vi "serial_cycle_thread.vi"() -> ()   [LabVIEW 2020]
doc: "该模板用于创建生产者／消费者模式的应用程序，以事件驱动的方式，生成队列中的项。如需通过响应事件实现代码的异步执行，同时不影响用户界面的响应速度，可考虑用该模式替代“用户界面事件处理器”模式。"
uses:
  <vilib>/Instr/_visa.llb/VISA Set IO Buffer Mask.ctl
  <vilib>/Instr/_visa.llb/VISA Configure Serial Port (Instr).vi
panel:
  in  "写入缓冲区":string="~\u00010000@SCNTRG1;\u0003"
  out "标准码词":string
  out "数据读取时间2":u32
  out "读取的数据":string
  in  "开等待(ms)2":u32
  in  "VISA资源名称2":refnum<visa-resource-name>
  in  "VISA资源名称 3":refnum<visa-resource-name>
  in  "开等待(ms)3":u32
  out "数据读取时间3":u32
  out "读取的数据3":string
  in  "开等待(ms)1":u32
  out "数据读取时间":u32
  out "读取的数据":string
  in  "VISA资源名称":refnum<visa-resource-name>
  in  "读取标准码词":bool
  in  "压缩机":bool
  in  "臭氧":bool
  in  "开始测试":bool
  in  "风机":bool
  in  "继电器调试":bool
  in  "打开开关":bool
  in  "串口资源":refnum<visa-resource-name>
  in  "stop":bool caption="停止"
  out "错误输出":errorcluster
  out "error out":errorcluster caption="继电器板错误输入输出"
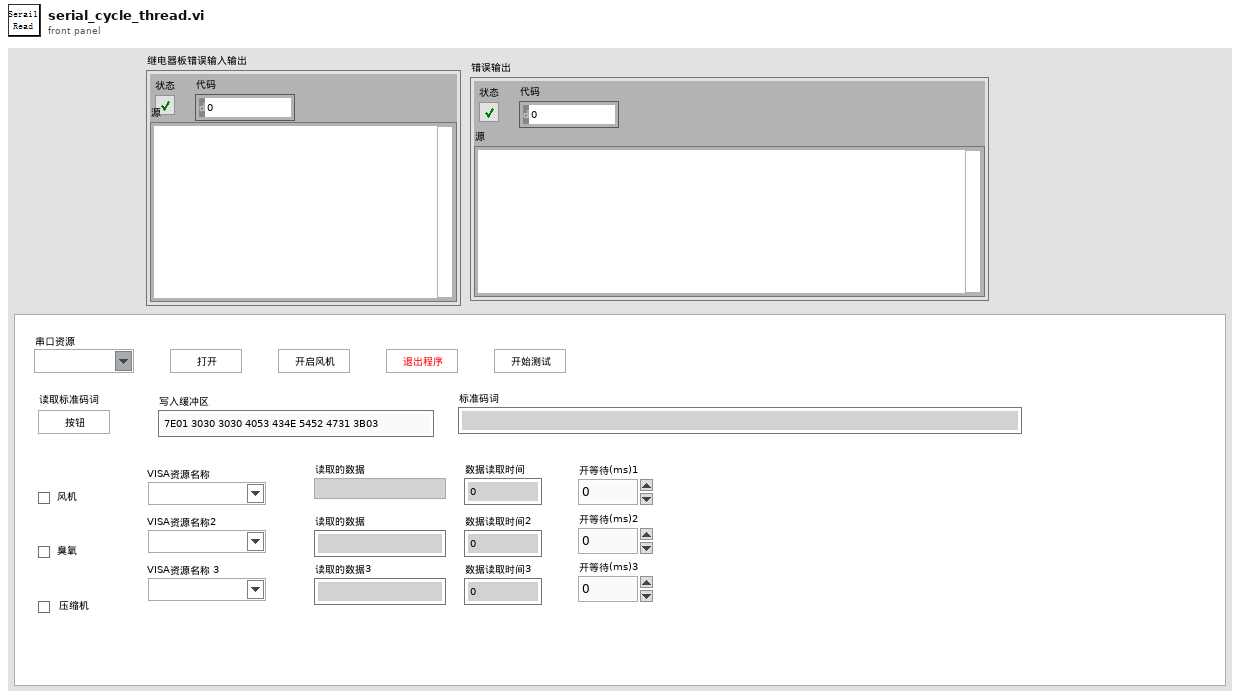
[diagram p1: front panel]
types:
  T1 = typedef "VISA Set IO Buffer Mask.ctl" = u16
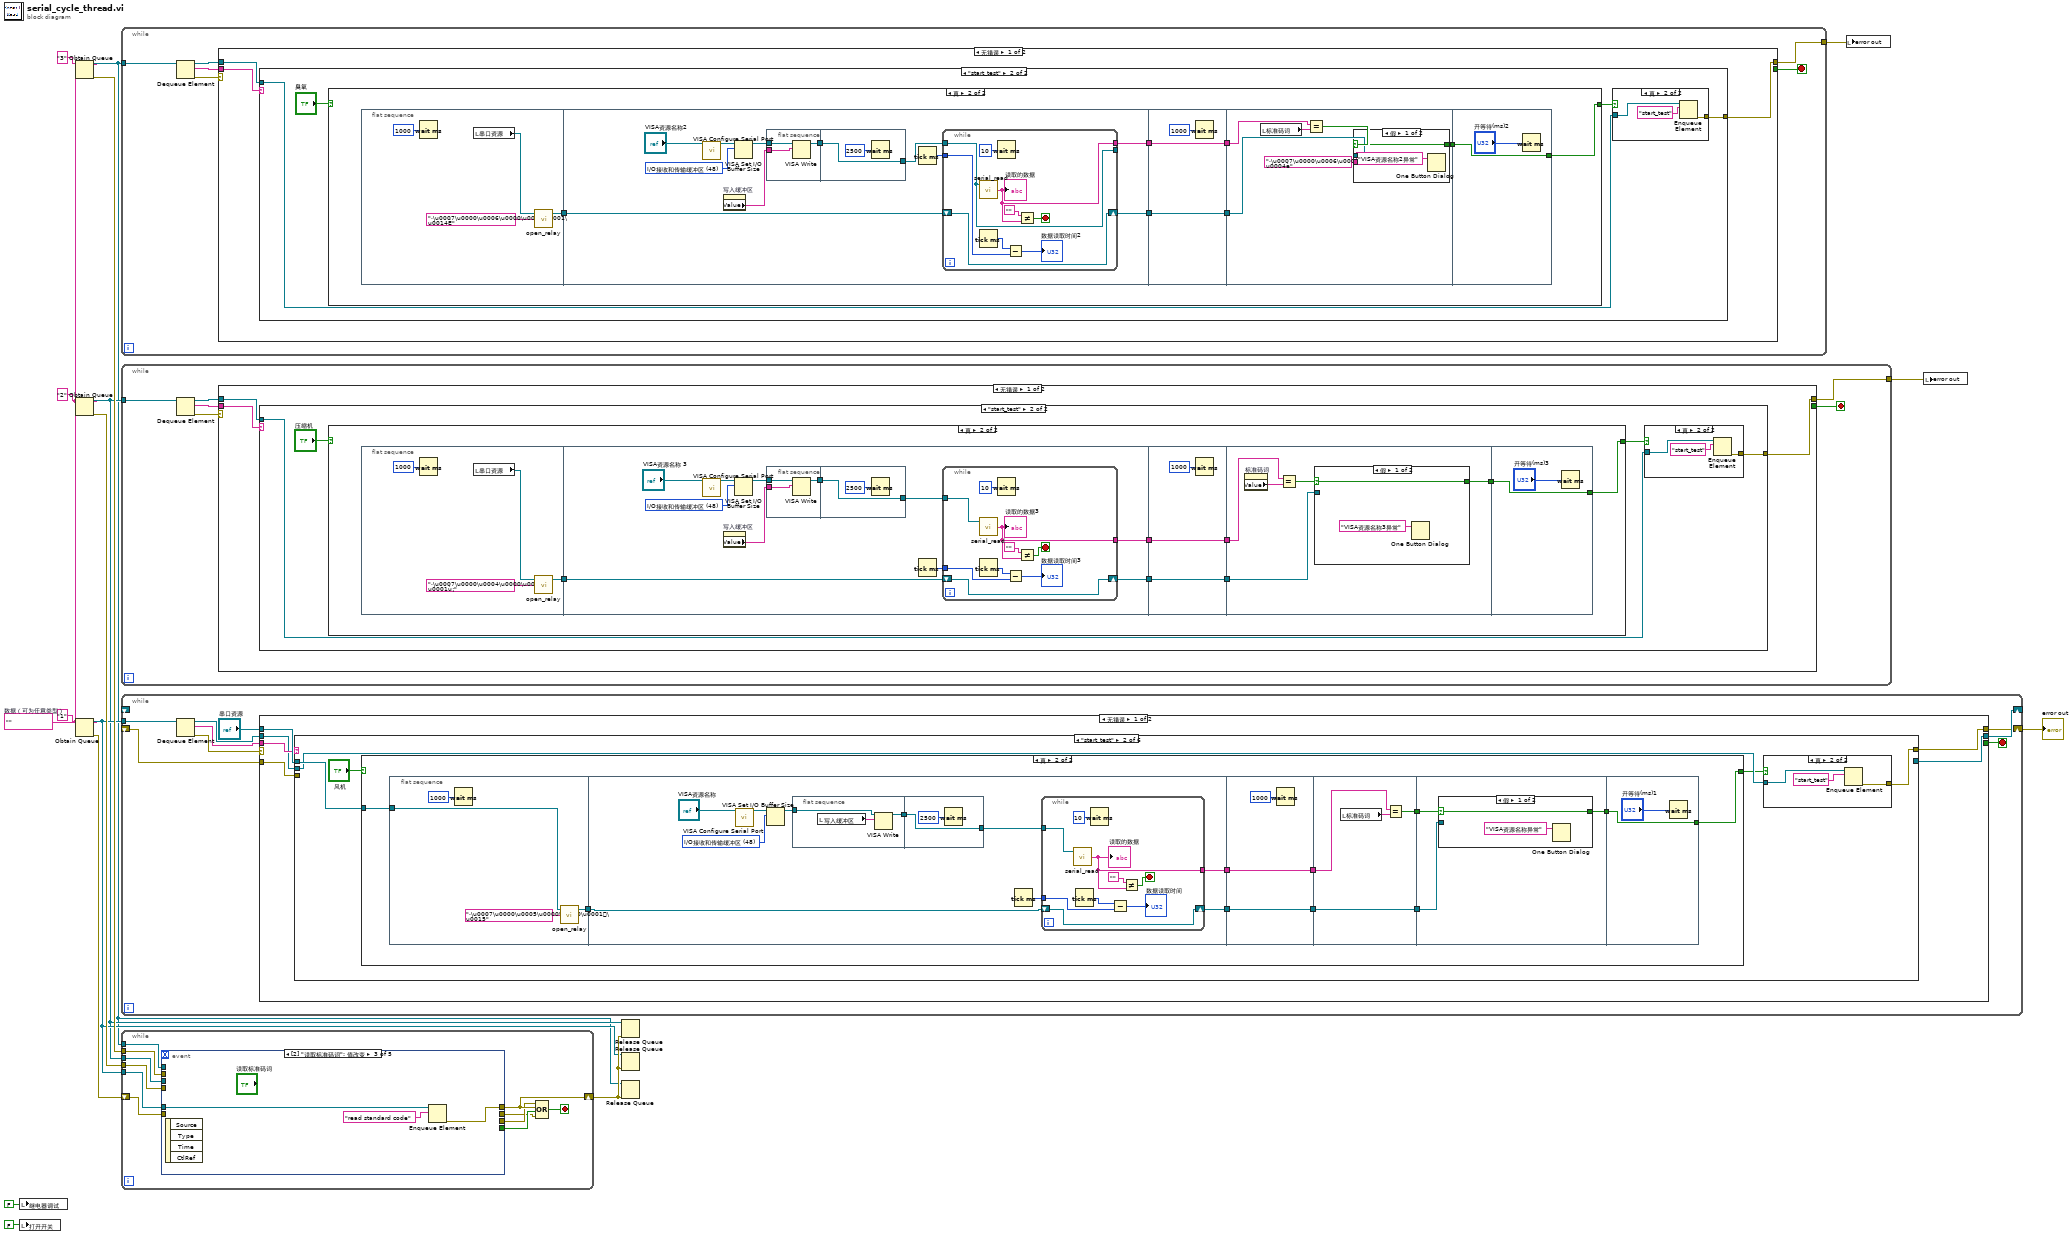
[diagram p0: block diagram]
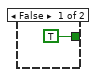
[diagram p4: hidden frame]
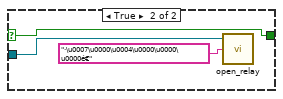
[diagram p5: hidden frame]
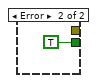
[diagram p6: hidden frame]
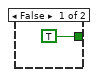
[diagram p9: hidden frame]
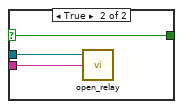
[diagram p10: hidden frame]
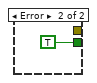
[diagram p11: hidden frame]
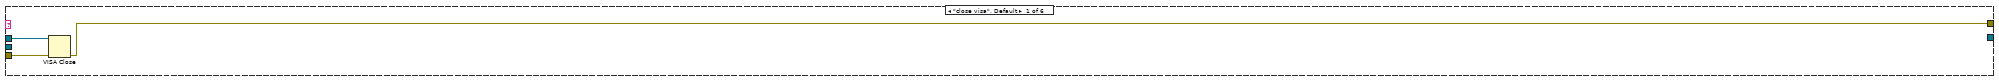
[diagram p12: hidden frame]
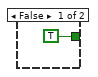
[diagram p14: hidden frame]
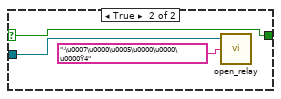
[diagram p15: hidden frame]
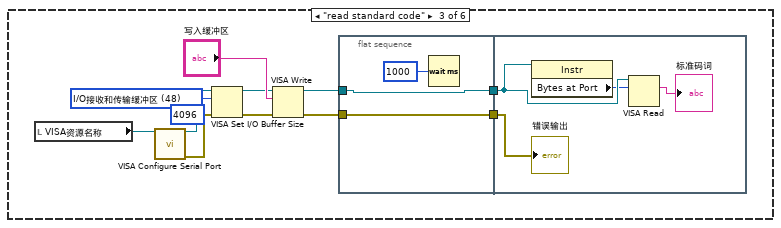
[diagram p16: hidden frame]
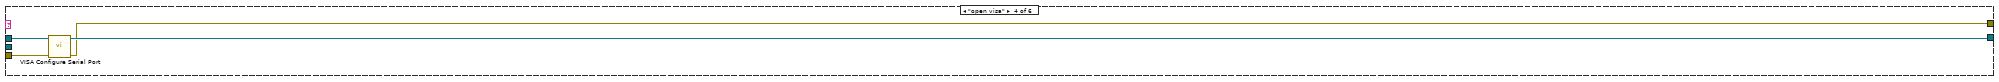
[diagram p17: hidden frame]
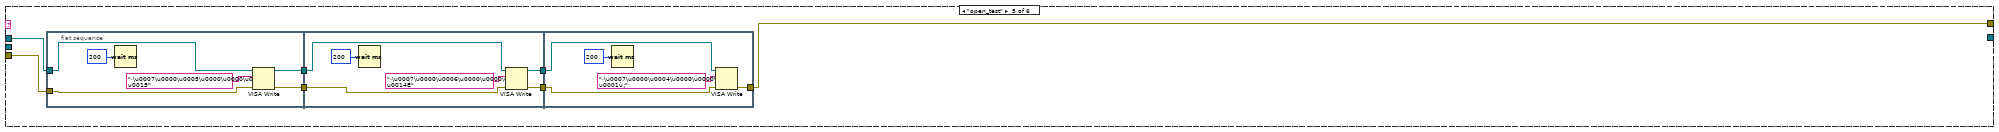
[diagram p18: hidden frame]
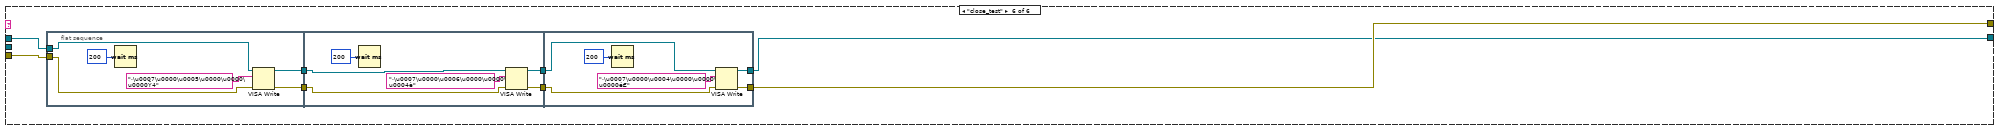
[diagram p19: hidden frame]
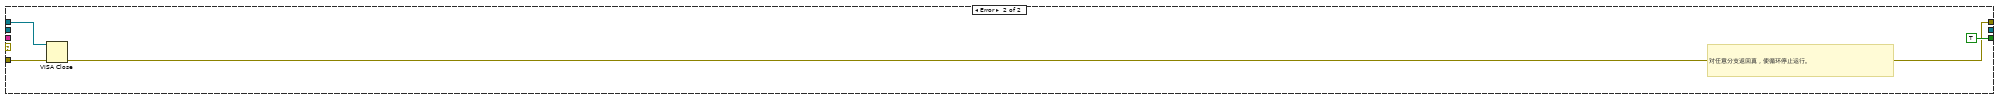
[diagram p20: hidden frame]
diagram:
  w12 = ""  # 数据（可为任意类型）
  n1 = local write "继电器调试"(FALSE ("继电器调试")) -> ()
  n2 = local write "打开开关"(FALSE ("打开开关")) -> ()
  n3 = Obtain Queue(name (unnamed)="3" ("名称（未命名）"), element data type=w12) -> (queue out=w3:refnum<queue>, error out=w11:errorcluster)  [unwired: 3 in, 1 out]
  n4 = Obtain Queue(name (unnamed)="2" ("名称（未命名）"), element data type=w12) -> (queue out=w4:refnum<queue>, error out=w10:errorcluster)  [unwired: 3 in, 1 out]
  n5 = Obtain Queue(name (unnamed)="1" ("名称（未命名）"), element data type=w12) -> (queue out=w8:refnum<queue>, error out=w16:errorcluster)  [unwired: 3 in, 1 out]
  n6 = while {
    tunnel: w3 -> [w19]
    tunnel: [w18] -> w1
    stop <- w20 stop-if-true
    n7 = Dequeue Element(queue=w19) -> (queue out=w17:refnum<queue>, element=w21:string, error out=w22:errorcluster)  [unwired: 2 in, 1 out]
    n8 = case shown="无错误" w22 {
      tunnel: w21 -> [w25 _]
      tunnel: [_ TRUE] -> w20
      tunnel: [w24 _] -> w18
      tunnel: w17 -> [w23 _]
      frame No Error {
        n9 = case shown="\"start_test\"" w25 {
          tunnel: [_ w27] -> w24
          tunnel: w23 -> [_ w26]
          frame "假", Default {
          }
          frame "start_test" {
            n10 = case shown="真" "臭氧" {
              tunnel: [TRUE w37] -> w28
              frame False {
              }
              frame True {
                n11 = flat-sequence {
                  tunnel: [w43] -> w40
                  tunnel: w40 -> [w55]
                  tunnel: [w54] -> w39
                  tunnel: [w45] -> w35
                  tunnel: w39 -> [w72]
                  tunnel: [w72] -> w38
                  tunnel: [w70] -> w36
                  tunnel: w35 -> [w70]
                  tunnel: w38 -> [w74]
                  tunnel: w36 -> [w78]
                  tunnel: [w73] -> w34
                  tunnel: [w84] -> w37
                  tunnel: w34 -> [w84]
                  frame #0 {
                    n12 = Wait (ms)(milliseconds to wait=u32 1000 ("等待时间（毫秒）")) -> ()  [unwired: 1 out]
                    n13 = local read "串口资源"() -> (w41:refnum<visa-resource-name>)
                    n14 = call "open_relay.vi"("写入缓冲区"="·\u0007\u0000\u0006\u0000\u0000\u0001\u0014É", "VISA资源名称"=w41) -> ("VISA资源名称输出"=w43:refnum<visa-resource-name>)  [unwired: 1 in, 2 out]
                  }
                  frame #1 {
                    w50 = T1 48 items=["I/O接收缓冲区"=16, "I/O传输缓冲区"=32, "I/O接收和传输缓冲区"=48] ("Mask")
                    n15 = call-poly "VISA Configure Serial Port"("VISA resource name"="VISA资源名称2") -> ("VISA resource name out"=w51:refnum<visa-resource-name>)  [unwired: 13 in, 1 out]
                    n16 = property on="写入缓冲区" class="Str"() -> ("Value"=w49:string)  [unwired: 2 in, 2 out]
                    n17 = VISA Set I/O Buffer Size(VISA resource name=w51, mask (16)=w50) -> (VISA resource name out=w48:refnum<visa-resource-name>)  [unwired: 2 in, 1 out]
                    n18 = flat-sequence {
                      tunnel: w49 -> [w58]
                      tunnel: w48 -> [w57]
                      tunnel: [w56] -> w46
                      tunnel: [w60] -> w47
                      tunnel: w46 -> [w60]
                      frame #0 {
                        n19 = VISA Write(VISA resource name=w57, write buffer=w58) -> (VISA resource name out=w56:refnum<visa-resource-name>)  [unwired: 1 in, 2 out]
                      }
                      frame #1 {
                        n20 = Wait (ms)(milliseconds to wait=u32 2500 ("等待时间（毫秒）")) -> ()  [unwired: 1 out]
                      }
                    }
                    n21 = Tick Count (ms)() -> (millisecond timer value=w53:u32)
                    n22 = while {
                      shift-right: [w66] -> w54
                      shift-left: w55 -> [w66]
                      tunnel: [w62] -> _
                      tunnel: w53 -> [w64]
                      tunnel: w47 -> [w62]
                      tunnel: [w61] -> w45
                      stop <- w68 stop-if-true
                      n23 = call "serial_read.vi"("VISA资源名称"=w62) -> ("读取缓冲区"=w61:string)  [unwired: 2 in, 2 out]
                      "读取的数据" <- w61
                      n24 = Tick Count (ms)() -> (millisecond timer value=w65:u32)
                      n25 = Wait (ms)(milliseconds to wait=u32 10 ("等待时间（毫秒）")) -> ()  [unwired: 1 out]
                      n26 = Subtract(x=w65, y=w64) -> (x-y=→"数据读取时间2":u32)
                      n27 = Not Equal?(x="", y=w61) -> (x != y?=w68:bool)
                    }
                  }
                  frame #2 {
                    n28 = Wait (ms)(milliseconds to wait=u32 1000 ("等待时间（毫秒）")) -> ()  [unwired: 1 out]
                  }
                  frame #3 {
                    n29 = local read "标准码词"() -> (w77:string)
                    n30 = Equal?(x=w78, y=w77) -> (x = y?=w76:bool)
                    n31 = case shown="假" w76 {
                      selector: w76 -> [w80 w81]
                      tunnel: "·\u0007\u0000\u0006\u0000\u0000\u0000\u0004è" ("写入缓冲区") -> [_ w83]
                      tunnel: w74 -> [_ w82]
                      tunnel: [w80 w81] -> w73
                      frame False {
                        n32 = One Button Dialog(message="VISA资源名称2异常" ("消息")) -> ()  [unwired: 1 in, 1 out]
                      }
                      frame True {
                        n33 = call "open_relay.vi"("写入缓冲区"=w83, "VISA资源名称"=w82) -> ()  [unwired: 1 in, 3 out]
                      }
                    }
                  }
                  frame #4 {
                    n34 = Wait (ms)(milliseconds to wait="开等待(ms)2") -> ()  [unwired: 1 out]
                  }
                }
              }
            }
            n35 = case shown="真" w28 {
              tunnel: [_ w31] -> w27
              tunnel: w26 -> [_ w30]
              frame False {
              }
              frame True {
                n36 = Enqueue Element(queue=w30, element="start_test" ("元素")) -> (error out=w31:errorcluster)  [unwired: 2 in, 2 out]
              }
            }
          }
        }
      }
      frame Error {
      }
    }
  }
  n37 = while {
    tunnel: w4 -> [w89]
    tunnel: [w88] -> w2
    stop <- w90 stop-if-true
    n38 = Dequeue Element(queue=w89) -> (queue out=w87:refnum<queue>, element=w91:string, error out=w92:errorcluster)  [unwired: 2 in, 1 out]
    n39 = case shown="无错误" w92 {
      tunnel: w91 -> [w95 _]
      tunnel: [_ TRUE] -> w90
      tunnel: [w94 _] -> w88
      tunnel: w87 -> [w93 _]
      frame No Error {
        n40 = case shown="\"start_test\"" w95 {
          tunnel: [_ w97] -> w94
          tunnel: w93 -> [_ w96]
          frame "假", Default {
          }
          frame "start_test" {
            n41 = case shown="真" "压缩机" {
              tunnel: [TRUE w107] -> w98
              frame False {
              }
              frame True {
                n42 = flat-sequence {
                  tunnel: [w113] -> w110
                  tunnel: w110 -> [w125]
                  tunnel: [w124] -> w109
                  tunnel: [w115] -> w105
                  tunnel: w109 -> [w142]
                  tunnel: [w142] -> w108
                  tunnel: [w140] -> w106
                  tunnel: w105 -> [w140]
                  tunnel: w108 -> [w144]
                  tunnel: w106 -> [w147]
                  tunnel: [w143] -> w104
                  tunnel: [w153] -> w107
                  tunnel: w104 -> [w153]
                  frame #0 {
                    n43 = Wait (ms)(milliseconds to wait=u32 1000 ("等待时间（毫秒）")) -> ()  [unwired: 1 out]
                    n44 = local read "串口资源"() -> (w111:refnum<visa-resource-name>)
                    n45 = call "open_relay.vi"("写入缓冲区"="·\u0007\u0000\u0004\u0000\u0000\u0001ù¡", "VISA资源名称"=w111) -> ("VISA资源名称输出"=w113:refnum<visa-resource-name>)  [unwired: 1 in, 2 out]
                  }
                  frame #1 {
                    w120 = T1 48 items=["I/O接收缓冲区"=16, "I/O传输缓冲区"=32, "I/O接收和传输缓冲区"=48] ("Mask")
                    n46 = call-poly "VISA Configure Serial Port"("VISA resource name"="VISA资源名称 3") -> ("VISA resource name out"=w121:refnum<visa-resource-name>)  [unwired: 13 in, 1 out]
                    n47 = property on="写入缓冲区" class="Str"() -> ("Value"=w117:string)  [unwired: 2 in, 2 out]
                    n48 = VISA Set I/O Buffer Size(VISA resource name=w121, mask (16)=w120) -> (VISA resource name out=w119:refnum<visa-resource-name>)  [unwired: 2 in, 1 out]
                    n49 = flat-sequence {
                      tunnel: w119 -> [w128]
                      tunnel: w117 -> [w126]
                      tunnel: [w127] -> w116
                      tunnel: [w130] -> w118
                      tunnel: w116 -> [w130]
                      frame #0 {
                        n50 = VISA Write(VISA resource name=w128, write buffer=w126) -> (VISA resource name out=w127:refnum<visa-resource-name>)  [unwired: 1 in, 2 out]
                      }
                      frame #1 {
                        n51 = Wait (ms)(milliseconds to wait=u32 2500 ("等待时间（毫秒）")) -> ()  [unwired: 1 out]
                      }
                    }
                    n52 = Tick Count (ms)() -> (millisecond timer value=w123:u32)
                    n53 = while {
                      shift-right: [w136] -> w124
                      shift-left: w125 -> [w136]
                      tunnel: w118 -> [w134]
                      tunnel: w123 -> [w133]
                      tunnel: [w131] -> w115
                      stop <- w138 stop-if-true
                      n54 = call "serial_read.vi"("VISA资源名称"=w134) -> ("读取缓冲区"=w131:string)  [unwired: 2 in, 2 out]
                      "读取的数据3" <- w131
                      n55 = Tick Count (ms)() -> (millisecond timer value=w135:u32)
                      n56 = Wait (ms)(milliseconds to wait=u32 10 ("等待时间（毫秒）")) -> ()  [unwired: 1 out]
                      n57 = Subtract(x=w135, y=w133) -> (x-y=→"数据读取时间3":u32)
                      n58 = Not Equal?(x="", y=w131) -> (x != y?=w138:bool)
                    }
                  }
                  frame #2 {
                    n59 = Wait (ms)(milliseconds to wait=u32 1000 ("等待时间（毫秒）")) -> ()  [unwired: 1 out]
                  }
                  frame #3 {
                    n60 = property on="标准码词" class="Str"() -> ("Value"=w146:string)  [unwired: 2 in, 2 out]
                    n61 = Equal?(x=w147, y=w146) -> (x = y?=w145:bool)
                    n62 = case shown="假" w145 {
                      selector: w145 -> [w149 w150]
                      tunnel: w144 -> [_ w151]
                      tunnel: [w149 w150] -> w143
                      frame False {
                        n63 = One Button Dialog(message="VISA资源名称3异常" ("消息")) -> ()  [unwired: 1 in, 1 out]
                      }
                      frame True {
                        n64 = call "open_relay.vi"("写入缓冲区"="·\u0007\u0000\u0004\u0000\u0000\u0000é€", "VISA资源名称"=w151) -> ()  [unwired: 1 in, 3 out]
                      }
                    }
                  }
                  frame #4 {
                    n65 = Wait (ms)(milliseconds to wait="开等待(ms)3") -> ()  [unwired: 1 out]
                  }
                }
              }
            }
            n66 = case shown="真" w98 {
              tunnel: [_ w101] -> w97
              tunnel: w96 -> [_ w100]
              frame False {
              }
              frame True {
                n67 = Enqueue Element(queue=w100, element="start_test" ("元素")) -> (error out=w101:errorcluster)  [unwired: 2 in, 2 out]
              }
            }
          }
        }
      }
      frame Error {
      }
    }
  }
  n68 = while {
    tunnel: w8 -> [w164]
    shift-right: [w160] -> _
    shift-left: _ -> [_]
    shift-right: [w159] -> w15
    shift-left: _ -> [w158]
    stop <- w163 stop-if-true
    n69 = Dequeue Element(queue=w164) -> (queue out=w156:refnum<queue>, element=w161:string, error out=w162:errorcluster)  [unwired: 2 in, 1 out]
    n70 = case shown="无错误" w162 {
      tunnel: [_ TRUE] -> w163
      tunnel: w161 -> [w166 _]
      tunnel: [w170 _] -> w160
      tunnel: "串口资源" -> [w169 w313]
      tunnel: [w167 w311] -> w159
      tunnel: w158 -> [w168 w312]
      tunnel: w156 -> [w165 _]
      frame No Error {
        n71 = case shown="\"start_test\"" w166 {
          tunnel: [_ _ _ w260 _ w290] -> w170
          tunnel: w169 -> [w173 w177 _ w257 w267 w291]
          tunnel: w168 -> [w172 _ _ w258 w265 w289]
          tunnel: [w171 w174 _ w259 w266 w292] -> w167
          tunnel: w165 -> [_ w176 _ _ _ _]
          frame "close visa", Default {
            n72 = VISA Close(VISA resource name=w173, error in (no error)=w172) -> (error out=w171:errorcluster)
          }
          frame "start_test" {
            n73 = case shown="真" "风机" {
              tunnel: w177 -> [_ w192]
              tunnel: [TRUE w191] -> w175
              frame False {
              }
              frame True {
                n74 = flat-sequence {
                  tunnel: w192 -> [w196]
                  tunnel: [w194] -> w190
                  tunnel: w190 -> [w206]
                  tunnel: [w205] -> w189
                  tunnel: [w198] -> w185
                  tunnel: w189 -> [w223]
                  tunnel: [w223] -> w188
                  tunnel: [w221] -> w186
                  tunnel: w185 -> [w221]
                  tunnel: w188 -> [w227]
                  tunnel: [w227] -> w187
                  tunnel: w186 -> [w226]
                  tunnel: [w224] -> w184
                  tunnel: w187 -> [w229]
                  tunnel: w184 -> [w230]
                  tunnel: [w228] -> w183
                  tunnel: [w236] -> w191
                  tunnel: w183 -> [w236]
                  frame #0 {
                    n75 = Wait (ms)(milliseconds to wait=u32 1000 ("等待时间（毫秒）")) -> ()  [unwired: 1 out]
                    n76 = call "open_relay.vi"("写入缓冲区"="·\u0007\u0000\u0005\u0000\u0000\u0001\u0015", "VISA资源名称"=w196) -> ("VISA资源名称输出"=w194:refnum<visa-resource-name>)  [unwired: 1 in, 2 out]
                  }
                  frame #1 {
                    w201 = T1 48 items=["I/O接收缓冲区"=16, "I/O传输缓冲区"=32, "I/O接收和传输缓冲区"=48] ("Mask")
                    n77 = call-poly "VISA Configure Serial Port"("VISA resource name"="VISA资源名称") -> ("VISA resource name out"=w200:refnum<visa-resource-name>)  [unwired: 13 in, 1 out]
                    n78 = VISA Set I/O Buffer Size(VISA resource name=w200, mask (16)=w201) -> (VISA resource name out=w199:refnum<visa-resource-name>)  [unwired: 2 in, 1 out]
                    n79 = flat-sequence {
                      tunnel: w199 -> [w208]
                      tunnel: [w209] -> w197
                      tunnel: [w211] -> w202
                      tunnel: w197 -> [w211]
                      frame #0 {
                        n80 = local read "写入缓冲区"() -> (w207:string)
                        n81 = VISA Write(VISA resource name=w208, write buffer=w207) -> (VISA resource name out=w209:refnum<visa-resource-name>)  [unwired: 1 in, 2 out]
                      }
                      frame #1 {
                        n82 = Wait (ms)(milliseconds to wait=u32 2500 ("return count")) -> ()  [unwired: 1 out]
                      }
                    }
                    n83 = Tick Count (ms)() -> (millisecond timer value=w203:u32)
                    n84 = while {
                      shift-right: [w217] -> w205
                      shift-left: w206 -> [w217]
                      tunnel: w203 -> [w214]
                      tunnel: w202 -> [w213]
                      tunnel: [w212] -> w198
                      stop <- w219 stop-if-true
                      n85 = call "serial_read.vi"("VISA资源名称"=w213) -> ("读取缓冲区"=w212:string)  [unwired: 2 in, 2 out]
                      "读取的数据" <- w212
                      n86 = Tick Count (ms)() -> (millisecond timer value=w216:u32)
                      n87 = Wait (ms)(milliseconds to wait=u32 10 ("等待时间（毫秒）")) -> ()  [unwired: 1 out]
                      n88 = Subtract(x=w216, y=w214) -> (x-y=→"数据读取时间":u32)
                      n89 = Not Equal?(x="", y=w212) -> (x != y?=w219:bool)
                    }
                  }
                  frame #2 {
                    n90 = Wait (ms)(milliseconds to wait=u32 1000 ("等待时间（毫秒）")) -> ()  [unwired: 1 out]
                  }
                  frame #3 {
                    n91 = local read "标准码词"() -> (w225:string)
                    n92 = Equal?(x=w226, y=w225) -> (x = y?=w224:bool)
                  }
                  frame #4 {
                    n93 = case shown="假" w230 {
                      selector: w230 -> [w232 w233]
                      tunnel: w229 -> [_ w234]
                      tunnel: [w232 w233] -> w228
                      frame False {
                        n94 = One Button Dialog(message="VISA资源名称异常" ("消息")) -> ()  [unwired: 1 in, 1 out]
                      }
                      frame True {
                        n95 = call "open_relay.vi"("写入缓冲区"="·\u0007\u0000\u0005\u0000\u0000\u0000Ÿ4", "VISA资源名称"=w234) -> ()  [unwired: 1 in, 3 out]
                      }
                    }
                  }
                  frame #5 {
                    n96 = Wait (ms)(milliseconds to wait="开等待(ms)1") -> ()  [unwired: 1 out]
                  }
                }
              }
            }
            n97 = case shown="真" w175 {
              tunnel: w176 -> [_ w180]
              tunnel: [_ w179] -> w174
              frame False {
              }
              frame True {
                n98 = Enqueue Element(queue=w180, element="start_test" ("元素")) -> (error out=w179:errorcluster)  [unwired: 2 in, 2 out]
              }
            }
          }
          frame "read standard code" {
            w239 = T1 48 items=["I/O接收缓冲区"=16, "I/O传输缓冲区"=32, "I/O接收和传输缓冲区"=48] ("Mask")
            n99 = local read "VISA资源名称"() -> (w249:refnum<visa-resource-name>)
            n100 = call-poly "VISA Configure Serial Port"("VISA resource name"=w249) -> ("VISA resource name out"=w243:refnum<visa-resource-name>, "error out"=w241:errorcluster)  [unwired: 13 in]
            n101 = VISA Set I/O Buffer Size(VISA resource name=w243, mask (16)=w239, size (4096)=u32 4096 ("大小(4096)"), error in (no error)=w241) -> (VISA resource name out=w242:refnum<visa-resource-name>, error out=w240:errorcluster)
            n102 = VISA Write(VISA resource name=w242, write buffer="写入缓冲区", error in (no error)=w240) -> (VISA resource name out=w246:refnum<visa-resource-name>, error out=w247:errorcluster)  [unwired: 1 out]
            n103 = flat-sequence {
              tunnel: w246 -> [w251]
              tunnel: w247 -> [w252]
              tunnel: [w252] -> w245
              tunnel: [w251] -> w244
              tunnel: w245 -> [w256]
              tunnel: w244 -> [w255]
              frame #0 {
                n104 = Wait (ms)(milliseconds to wait=u32 1000 ("等待时间（毫秒）")) -> ()  [unwired: 1 out]
              }
              frame #1 {
                n105 = property class="Instr"(reference=w255) -> ("Bytes at Port"=w254:u32)  [unwired: 1 in, 2 out]
                n106 = VISA Read(VISA resource name=w255, byte count=w254) -> (read buffer=→"标准码词":string)  [unwired: 1 in, 3 out]
                "错误输出" <- w256
              }
            }
          }
          frame "open visa" {
            n107 = call-poly "VISA Configure Serial Port"("VISA resource name"=w257, "error in (no error)"=w258) -> ("VISA resource name out"=w260:refnum<visa-resource-name>, "error out"=w259:errorcluster)  [unwired: 12 in]
          }
          frame "open_test" {
            n108 = flat-sequence {
              tunnel: w267 -> [w273]
              tunnel: w265 -> [w270]
              tunnel: [w271] -> w264
              tunnel: [w269] -> w262
              tunnel: w264 -> [w279]
              tunnel: [w278] -> w263
              tunnel: w262 -> [w277]
              tunnel: [w276] -> w261
              tunnel: [w283] -> w266
              tunnel: w263 -> [w284]
              tunnel: w261 -> [w282]
              frame #0 {
                n109 = Wait (ms)(milliseconds to wait=u32 200 ("等待时间（毫秒）")) -> ()  [unwired: 1 out]
                n110 = VISA Write(VISA resource name=w273, write buffer="·\u0007\u0000\u0005\u0000\u0000\u0001\u0015" ("写入缓冲区"), error in (no error)=w270) -> (VISA resource name out=w269:refnum<visa-resource-name>, error out=w271:errorcluster)  [unwired: 1 out]
              }
              frame #1 {
                n111 = Wait (ms)(milliseconds to wait=u32 200 ("等待时间（毫秒）")) -> ()  [unwired: 1 out]
                n112 = VISA Write(VISA resource name=w277, write buffer="·\u0007\u0000\u0006\u0000\u0000\u0001\u0014É" ("写入缓冲区"), error in (no error)=w279) -> (VISA resource name out=w276:refnum<visa-resource-name>, error out=w278:errorcluster)  [unwired: 1 out]
              }
              frame #2 {
                n113 = Wait (ms)(milliseconds to wait=u32 200 ("等待时间（毫秒）")) -> ()  [unwired: 1 out]
                n114 = VISA Write(VISA resource name=w282, write buffer="·\u0007\u0000\u0004\u0000\u0000\u0001ù¡" ("写入缓冲区"), error in (no error)=w284) -> (error out=w283:errorcluster)  [unwired: 2 out]
              }
            }
          }
          frame "close_test" {
            n115 = flat-sequence {
              tunnel: w291 -> [w296]
              tunnel: w289 -> [w294]
              tunnel: [w298] -> w288
              tunnel: [w295] -> w287
              tunnel: w288 -> [w302]
              tunnel: w287 -> [w304]
              tunnel: [w303] -> w286
              tunnel: [w301] -> w285
              tunnel: [w310] -> w290
              tunnel: [w307] -> w292
              tunnel: w286 -> [w309]
              tunnel: w285 -> [w308]
              frame #0 {
                n116 = Wait (ms)(milliseconds to wait=u32 200 ("等待时间（毫秒）")) -> ()  [unwired: 1 out]
                n117 = VISA Write(VISA resource name=w296, write buffer="·\u0007\u0000\u0005\u0000\u0000\u0000Ÿ4" ("写入缓冲区"), error in (no error)=w294) -> (VISA resource name out=w295:refnum<visa-resource-name>, error out=w298:errorcluster)  [unwired: 1 out]
              }
              frame #1 {
                n118 = Wait (ms)(milliseconds to wait=u32 200 ("等待时间（毫秒）")) -> ()  [unwired: 1 out]
                n119 = VISA Write(VISA resource name=w304, write buffer="·\u0007\u0000\u0006\u0000\u0000\u0000\u0004è" ("写入缓冲区"), error in (no error)=w302) -> (VISA resource name out=w303:refnum<visa-resource-name>, error out=w301:errorcluster)  [unwired: 1 out]
              }
              frame #2 {
                n120 = Wait (ms)(milliseconds to wait=u32 200 ("等待时间（毫秒）")) -> ()  [unwired: 1 out]
                n121 = VISA Write(VISA resource name=w309, write buffer="·\u0007\u0000\u0004\u0000\u0000\u0000é€" ("写入缓冲区"), error in (no error)=w308) -> (VISA resource name out=w310:refnum<visa-resource-name>, error out=w307:errorcluster)  [unwired: 1 out]
              }
            }
          }
        }
      }
      frame Error {
        # "对任意分支返回真，使循环停止运行。"
        n122 = VISA Close(VISA resource name=w313, error in (no error)=w312) -> (error out=w311:errorcluster)
      }
    }
  }
  "error out" <- w15
  n123 = while {
    shift-right: [w322] -> w9
    shift-left: w16 -> [w324]
    tunnel: w8 -> [w325]
    tunnel: w11 -> [w319]
    tunnel: w10 -> [w317]
    tunnel: w3 -> [w316]
    tunnel: w4 -> [w315]
    stop <- w321 stop-if-true
    n124 = event shown="[2] \"读取标准码词\": 值改变" {
      selector: _ -> [_ _ _ _ _]
      dyn-events: _ -> [_ _ _ _ _]
      timeout: _ -> [_ _ _ _ _]
      tunnel: w325 -> [w330 w335 w341 w349 _]
      tunnel: w324 -> [w329 _ _ w346 w355]
      tunnel: [w328 w336 w340 w350 w355] -> w322
      tunnel: [_ _ _ _ "stop"] -> w323
      tunnel: [_ _ _ w343 w354] -> w320
      tunnel: w319 -> [_ _ _ _ w354]
      tunnel: [_ _ _ w344 w353] -> w318
      tunnel: w317 -> [_ _ _ _ w353]
      tunnel: w316 -> [_ _ _ w347 _]
      tunnel: w315 -> [_ _ _ w345 _]
      event "打开开关": Value Change {
        n125 = event-data() -> ()  [unwired: 1 in, 1 out]
        n126 = case shown="假" "打开开关" {
          tunnel: ["close visa" ("element") "open visa" ("element")] -> w326
          frame False {
          }
          frame True {
          }
        }
        n127 = Enqueue Element(queue=w330, element=w326, error in (no error)=w329) -> (error out=w328:errorcluster)  [unwired: 1 in, 2 out]
      }
      event "继电器调试": Value Change {
        n128 = event-data() -> ()  [unwired: 1 in, 3 out]
        n129 = case shown="假" "继电器调试" {
          tunnel: ["close_test" ("元素") "open_test" ("元素")] -> w333
          frame False {
          }
          frame True {
          }
        }
        n130 = Enqueue Element(queue=w335, element=w333) -> (error out=w336:errorcluster)  [unwired: 2 in, 2 out]
      }
      event "读取标准码词": Value Change {
        n131 = event-data() -> ()  [unwired: 1 in, 4 out]
        n132 = Enqueue Element(queue=w341, element="read standard code" ("元素")) -> (error out=w340:errorcluster)  [unwired: 2 in, 2 out]
      }
      event "开始测试": Value Change {
        n133 = event-data() -> ()  [unwired: 1 in, 4 out]
        n134 = case shown="真" "开始测试" {
          tunnel: ["stop_test" ("元素") "start_test" ("元素")] -> w342
          frame False {
          }
          frame True {
          }
        }
        n135 = Enqueue Element(queue=w349, element=w342, error in (no error)=w346) -> (error out=w350:errorcluster)  [unwired: 1 in, 2 out]
        n136 = Enqueue Element(queue=w347, element=w342) -> (error out=w344:errorcluster)  [unwired: 2 in, 2 out]
        n137 = Enqueue Element(queue=w345, element=w342) -> (error out=w343:errorcluster)  [unwired: 2 in, 2 out]
      }
      event "stop": Value Change {
        n138 = event-data() -> ()  [unwired: 1 in, 1 out]
      }
    }
    n139 = Compound Arithmetic op=OR ("复合运算")(w320, w322, w323, w318) -> (w321:bool)
  }
  n140 = Release Queue(queue=w4, error in (no error)=w9) -> ()  [unwired: 1 in, 3 out]
  n141 = Release Queue(queue=w8, error in (no error)=w9) -> ()  [unwired: 1 in, 3 out]
  n142 = Release Queue(queue=w3, error in (no error)=w9) -> ()  [unwired: 1 in, 3 out]
  n143 = local write "error out"(w1) -> ()
  n144 = local write "error out"(w2) -> ()
